vi "GetNearestImplemention.vi"(8 "error in (no error)":errorcluster, 11 "SubVI in":refnum<vi>) -> (3 "output string":string)   [LabVIEW 2017]
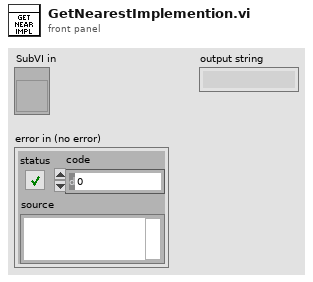
[diagram p1: front panel]
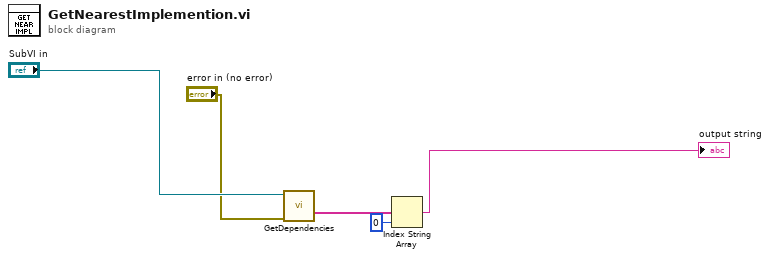
[diagram p0: block diagram]
diagram:
  n1 = call "GetDependencies.vi"("error in (no error)"="error in (no error)", "SubVI in"="SubVI in") -> ("Dependency Names"=w3:string[])  [unwired: 6 in, 3 out]
  n2 = Index String Array(1:0 ("index"), 2:w3) -> (0:→"output string":string)  [unwired: 1 in]
